vi "_builtins_visibles_reset.vi"(8 "error in (no error)":errorcluster, 10 "Reset Visible":T1(array[cluster]), 11 "GObjects in":refnum<vi>[](array[refnum])) -> (0 "error out":errorcluster, 3 "GObjects out":refnum<vi>[](array[refnum]))   [LabVIEW 2019, in "Script.lvlib"]
doc: "Resets the visible objects of the GObjects.\n\nCreated by: Ryan Pacini"
uses:
  Script.lvlib
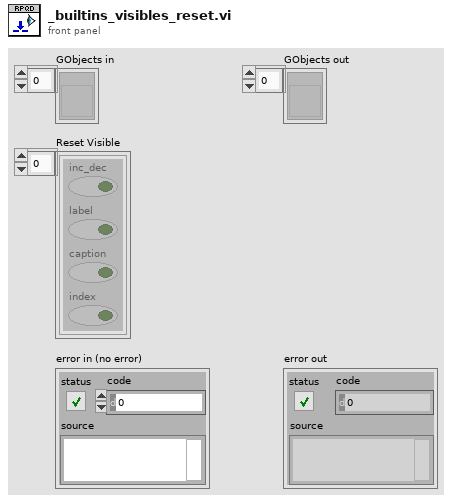
[diagram p1: front panel]
types:
  T1 = cluster{"inc_dec":bool, "label":bool, "caption":bool, "index":bool}[]
  T2 = cluster{"inc_dec":bool, "label":bool, "caption":bool, "index":bool}
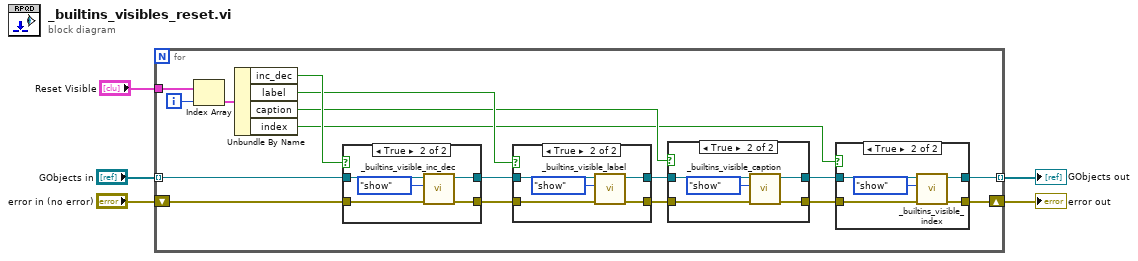
[diagram p0: block diagram]
diagram:
  n1 = for {
    tunnel: "GObjects in" -> [w21] mode=indexing
    shift-right: [w7] -> w3
    shift-left: "error in (no error)" -> [w22]
    tunnel: [w9] -> w2 mode=indexing
    tunnel: "Reset Visible" -> [w16]
    i -> [w15]
    n2 = Index Array(array=w16, index=w15) -> (element=w14:T2)
    n3 = Unbundle By Name(w14) -> ("inc_dec"=w13:bool, "label"=w12:bool, "caption"=w11:bool, "index"=w6:bool)
    n4 = case shown="True" w13 {
      tunnel: w22 -> [w44 w50]
      tunnel: w21 -> [w45 w49]
      tunnel: [w45 w47] -> w18
      tunnel: [w44 w46] -> w17
      frame False {
      }
      frame True {
        n5 = call "_builtins_visible_inc_dec.vi"("error in (no error)"=w50, "inc/dec"=enum8{"hide", "show"}."show", "GObject in"=w49) -> ("error out"=w46:errorcluster, "GObject out"=w47:refnum<vi>)  [unwired: 5 in, 2 out]
      }
    }
    n6 = case shown="True" w12 {
      tunnel: [w38 w43] -> w20
      tunnel: [w37 w42] -> w19
      tunnel: w18 -> [w38 w41]
      tunnel: w17 -> [w37 w40]
      frame False {
      }
      frame True {
        n7 = call "_builtins_visible_label.vi"("error in (no error)"=w40, "label"=enum8{"hide", "show"}."show", "GObject in"=w41) -> ("error out"=w42:errorcluster, "GObject out"=w43:refnum<vi>)  [unwired: 5 in, 2 out]
      }
    }
    n8 = case shown="True" w11 {
      tunnel: w20 -> [w31 w36]
      tunnel: w19 -> [w30 w35]
      tunnel: [w30 w34] -> w8
      tunnel: [w31 w33] -> w10
      frame False {
      }
      frame True {
        n9 = call "_builtins_visible_caption.vi"("error in (no error)"=w35, "caption"=enum8{"hide", "show"}."show", "GObject in"=w36) -> ("error out"=w34:errorcluster, "GObject out"=w33:refnum<vi>)  [unwired: 5 in, 2 out]
      }
    }
    n10 = case shown="True" w6 {
      tunnel: w10 -> [w24 w29]
      tunnel: [w24 w28] -> w9
      tunnel: w8 -> [w23 w27]
      tunnel: [w23 w26] -> w7
      frame False {
      }
      frame True {
        n11 = call "_builtins_visible_index.vi"("error in (no error)"=w27, "index display"=enum8{"hide", "show"}."show", "GObject in"=w29) -> ("error out"=w26:errorcluster, "GObject out"=w28:refnum<vi>)  [unwired: 5 in, 2 out]
      }
    }
  }
  "GObjects out" <- w2
  "error out" <- w3
